vi "Standalone DAQ IO Config UI.vi"() -> ()   [LabVIEW 2022 SP3, in "DAQ.lvclass"]
doc: "Developed by Kevin Thompson\nkevin@thompsonengineering.net\n\nCopyright 2018-2020\nThompson Engineering, LLC"
uses:
  DAQ.lvclass
  DataTypes/TD DI Config--cluster.ctl
  DataTypes/TD DI Task--cluster.ctl
  DataTypes/TD DI Channel--cluster.ctl
  DataTypes/TD DO Config--cluster.ctl
  DataTypes/TD DO Channel--cluster.ctl
  DataTypes/TD AI Config--cluster.ctl
  DataTypes/TD AI Task--cluster.ctl
  DataTypes/TD AI Channel--cluster.ctl
  DataTypes/TD DataValueConversion--cluster.ctl
  DataTypes/TD AI DAQ Type--enum.ctl
  DataTypes/TD AI Force Bridge--cluster.ctl
  DataTypes/TD AO Config--cluster.ctl
  DataTypes/TD AO Channel--cluster.ctl
  DataTypes/TD IO Node Definition--cluster.ctl
panel:
  in  "IO Nodes":T1 {"AO Config"."AO Channels"."Conversion"."ScaleOffset" format="%.3f"; "AO Config"."AO Channels"."Conversion"."MinEngUnit" format="%.3f"; "AO Config"."AO Channels"."Conversion"."MaxEngUnit" format="%.3f"; "AO Config"."AO Channels"."Conversion"."MinSignal" format="%.3f"; "AO Config"."AO Channels"."Conversion"."MaxSignal" format="%.3f"; "AI Config"."AI Tasks"."AI Channels"."Conversion"."ScaleOffset" format="%.3f"; "AI Config"."AI Tasks"."AI Channels"."Conversion"."MinEngUnit" format="%.3f"; "AI Config"."AI Tasks"."AI Channels"."Conversion"."MaxEngUnit" format="%.3f"; "AI Config"."AI Tasks"."AI Channels"."Conversion"."MinSignal" format="%.3f"; "AI Config"."AI Tasks"."AI Channels"."Conversion"."MaxSignal" format="%.3f"; "AI Config"."AI Tasks"."AI Channels"."Terminal Configuration" items=["default"=-1, "RSE"=10083, "NRSE"=10078, "Differential"=10106, "Pseudodifferential"=12529]}
  in  "LoadFile":bool
  in  "Config File":path
  in  "ApplyAll":bool
  out "Error":bool
  in  "Exit":bool
  in  "SaveAll":bool
  out "Tab Control":T15(tab)
  in  "DI Config":T2
  in  "DO Config":T5
  in  "AI Config":T7 {"AI Tasks"."AI Channels"."Force Bridge"."scaling information"."physical units" items=["Newtons"=15875, "Pounds"=15876, "kgf"=15877]; "AI Tasks"."AI Channels"."Force Bridge"."scaling information"."electrical units" items=["Volts/Volt"=15896, "mVolts/Volt"=15897]; "AI Tasks"."AI Channels"."Force Bridge"."bridge information"."voltage excitation source" items=["Internal"=10200, "External"=10167]; "AI Tasks"."AI Channels"."Force Bridge"."bridge information"."bridge configuration" items=["Full Bridge"=10182, "Half Bridge"=10187, "Quarter Bridge"=10270]; "AI Tasks"."AI Channels"."Conversion"."ScaleOffset" format="%.3f"; "AI Tasks"."AI Channels"."Conversion"."MinEngUnit" format="%.3f"; "AI Tasks"."AI Channels"."Conversion"."MaxEngUnit" format="%.3f"; "AI Tasks"."AI Channels"."Conversion"."MinSignal" format="%.3f"; "AI Tasks"."AI Channels"."Conversion"."MaxSignal" format="%.3f"; "AI Tasks"."AI Channels"."Terminal Configuration" items=["default"=-1, "RSE"=10083, "NRSE"=10078, "Differential"=10106, "Pseudodifferential"=12529]}
  in  "AO Config":T13 {"AO Channels"."Conversion"."ScaleOffset" format="%.3f"; "AO Channels"."Conversion"."MinEngUnit" format="%.3f"; "AO Channels"."Conversion"."MaxEngUnit" format="%.3f"; "AO Channels"."Conversion"."MinSignal" format="%.3f"; "AO Channels"."Conversion"."MaxSignal" format="%.3f"}
  in  "ConfigSections":i32(listbox)
  # "D A Q   I O   C O N F I G   U T I L I T Y"
  # "* Application Restart Required"
  # "DI Config"
  # "DO Config"
  # "AI Config"
  # "AO Config"
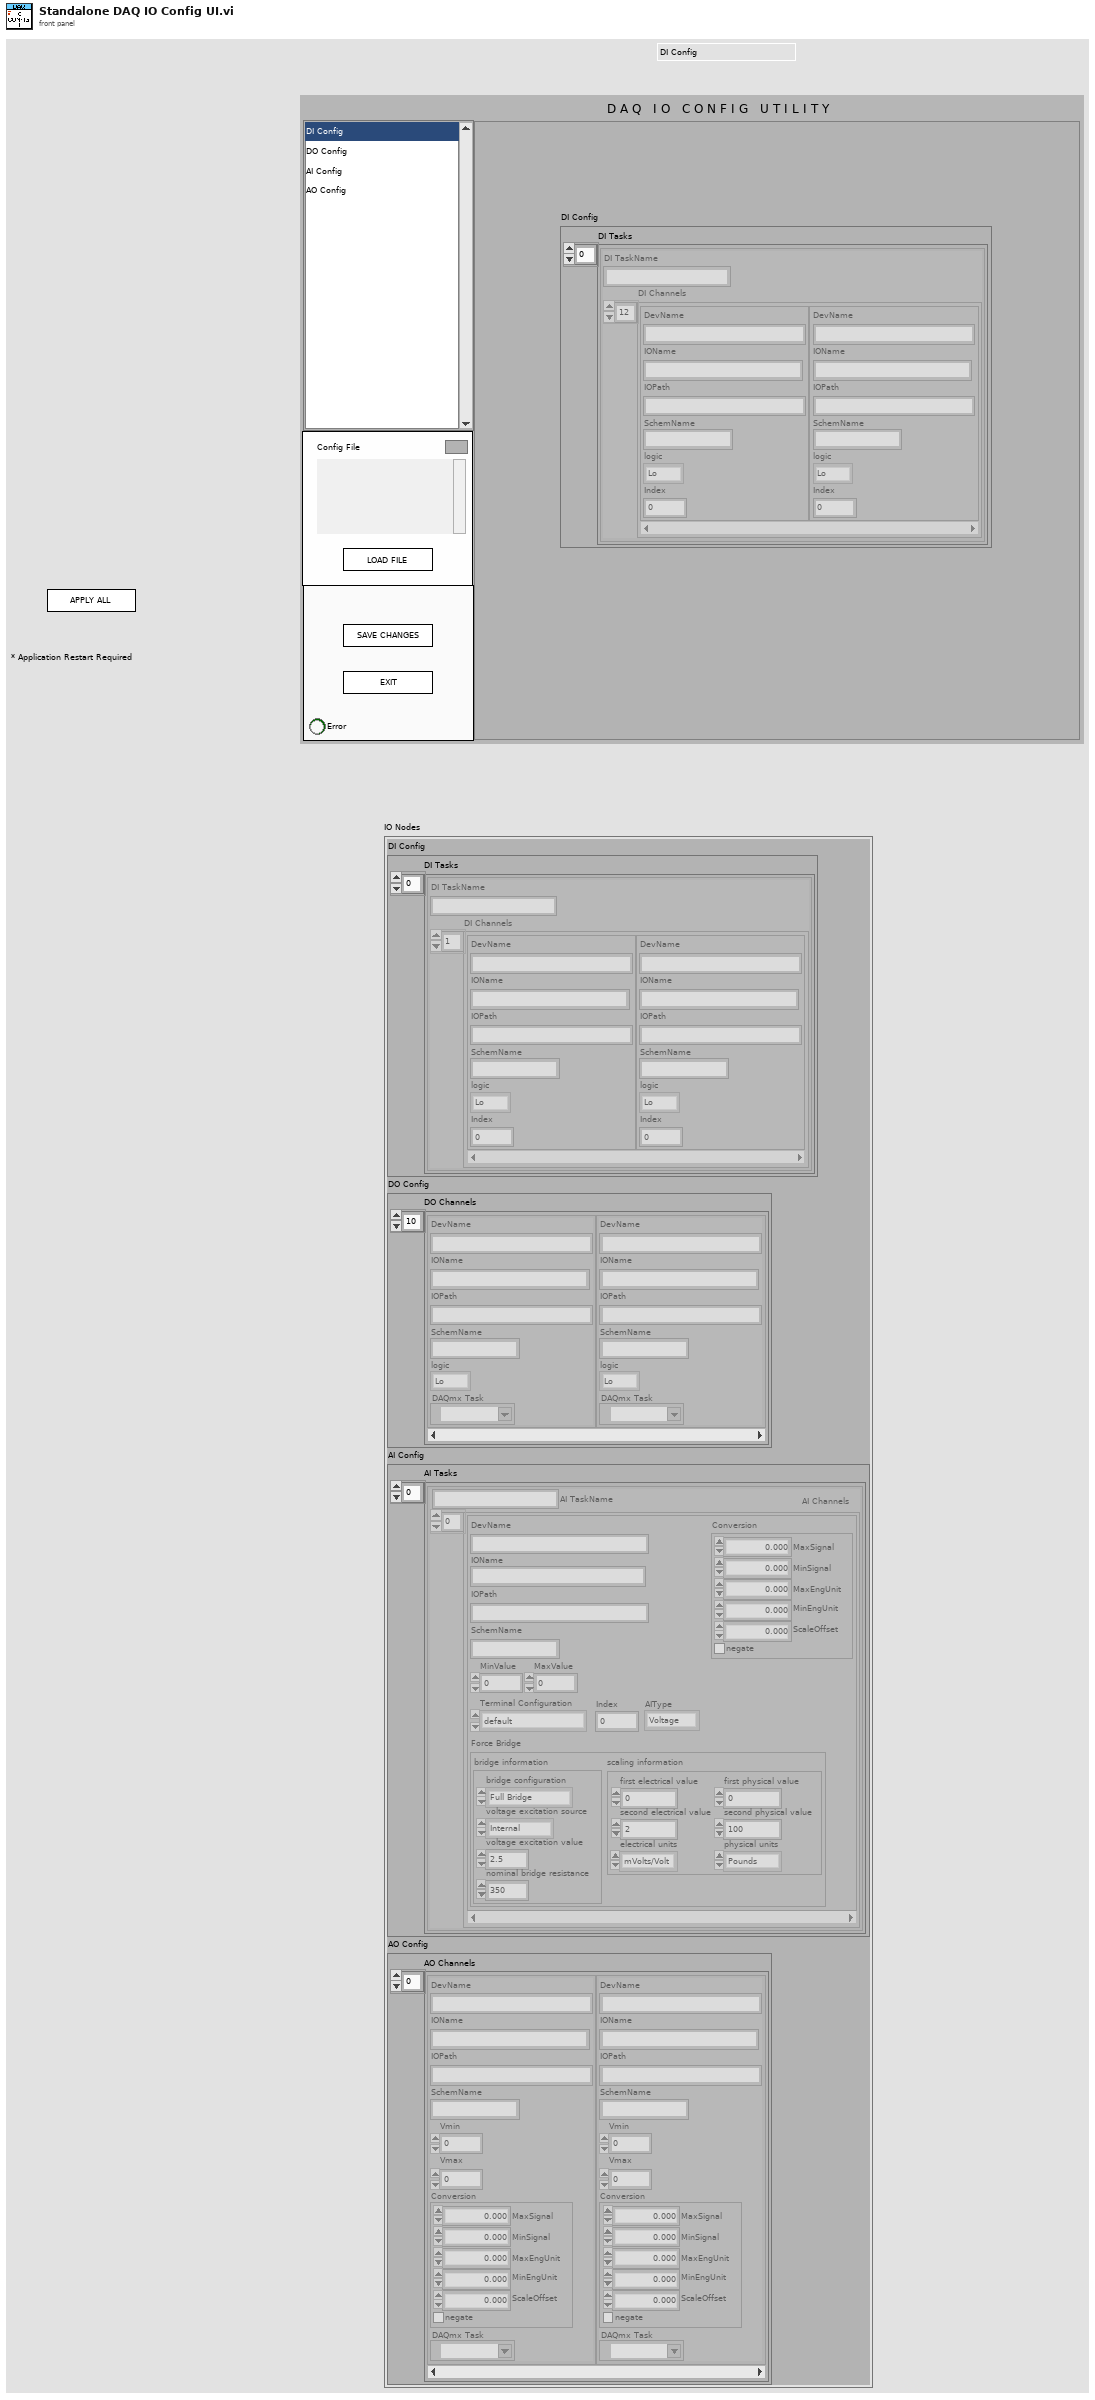
[diagram p1: front panel]
types:
  T1 = typedef "DAQ.lvclass/TD IO Node Definition--cluster.ctl" = cluster{"DI Config":T2, "DO Config":T5, "AI Config":T7, "AO Config":T13}
  T2 = typedef "DAQ.lvclass/TD DI Config--cluster.ctl" = cluster{"DI Tasks":T3[]}
  T3 = typedef "DAQ.lvclass/TD DI Task--cluster.ctl" = cluster{"DI TaskName":string, "DI Channels":T4[]}
  T4 = typedef "DAQ.lvclass/TD DI Channel--cluster.ctl" = cluster{"DevName":string, "IOName":string, "IOPath":string, "SchemName":string, "logic":enum16{"Lo", "Hi"}, "Index":i32}
  T5 = typedef "DAQ.lvclass/TD DO Config--cluster.ctl" = cluster{"DO Channels":T6[]}
  T6 = typedef "DAQ.lvclass/TD DO Channel--cluster.ctl" = cluster{"DevName":string, "IOName":string, "IOPath":string, "SchemName":string, "logic":enum16{"Lo", "Hi"}, "DAQmx Task":refnum<k21>}
  T7 = typedef "DAQ.lvclass/TD AI Config--cluster.ctl" = cluster{"AI Tasks":T8[]}
  T8 = typedef "DAQ.lvclass/TD AI Task--cluster.ctl" = cluster{"AI TaskName":string, "AI Channels":T9[]}
  T9 = typedef "DAQ.lvclass/TD AI Channel--cluster.ctl" = cluster{"DevName":string, "IOName":string, "IOPath":string, "SchemName":string, "MinValue":dbl, "MaxValue":dbl, "Terminal Configuration":i32, "Index":i32, "Conversion":T10, "AIType":T11, "Force Bridge":T12}
  T10 = typedef "DAQ.lvclass/TD DataValueConversion--cluster.ctl" = cluster{"MaxSignal":dbl, "MinSignal":dbl, "MaxEngUnit":dbl, "MinEngUnit":dbl, "ScaleOffset":dbl, "negate":bool}
  T11 = typedef "DAQ.lvclass/TD AI DAQ Type--enum.ctl" = enum16{"Voltage", "Current", "Strain Gage", "Force Bridge"}
  T12 = typedef "DAQ.lvclass/TD AI Force Bridge--cluster.ctl" = cluster{"bridge information":cluster{"bridge configuration":i32, "voltage excitation source":i32, "voltage excitation value":dbl, "nominal bridge resistance":dbl}, "scaling information":cluster{"first electrical value":dbl, "second electrical value":dbl, "electrical units":i32, "first physical value":dbl, "second physical value":dbl, "physical units":i32}}
  T13 = typedef "DAQ.lvclass/TD AO Config--cluster.ctl" = cluster{"AO Channels":T14[]}
  T14 = typedef "DAQ.lvclass/TD AO Channel--cluster.ctl" = cluster{"DevName":string, "IOName":string, "IOPath":string, "SchemName":string, "Vmin":dbl, "Vmax":dbl, "Conversion":T10, "DAQmx Task":refnum<k21>}
  T15 = enum32{"DI Config", "DO Config", "AI Config", "AO Config"}
  T16 = enum32{"Invalid", "Default", "Floating", "Floating/Auto-Hide", "Modal"}
  T17 = enum32{"Invalid", "Standard", "Closed", "Hidden", "Minimized", "Maximized"}
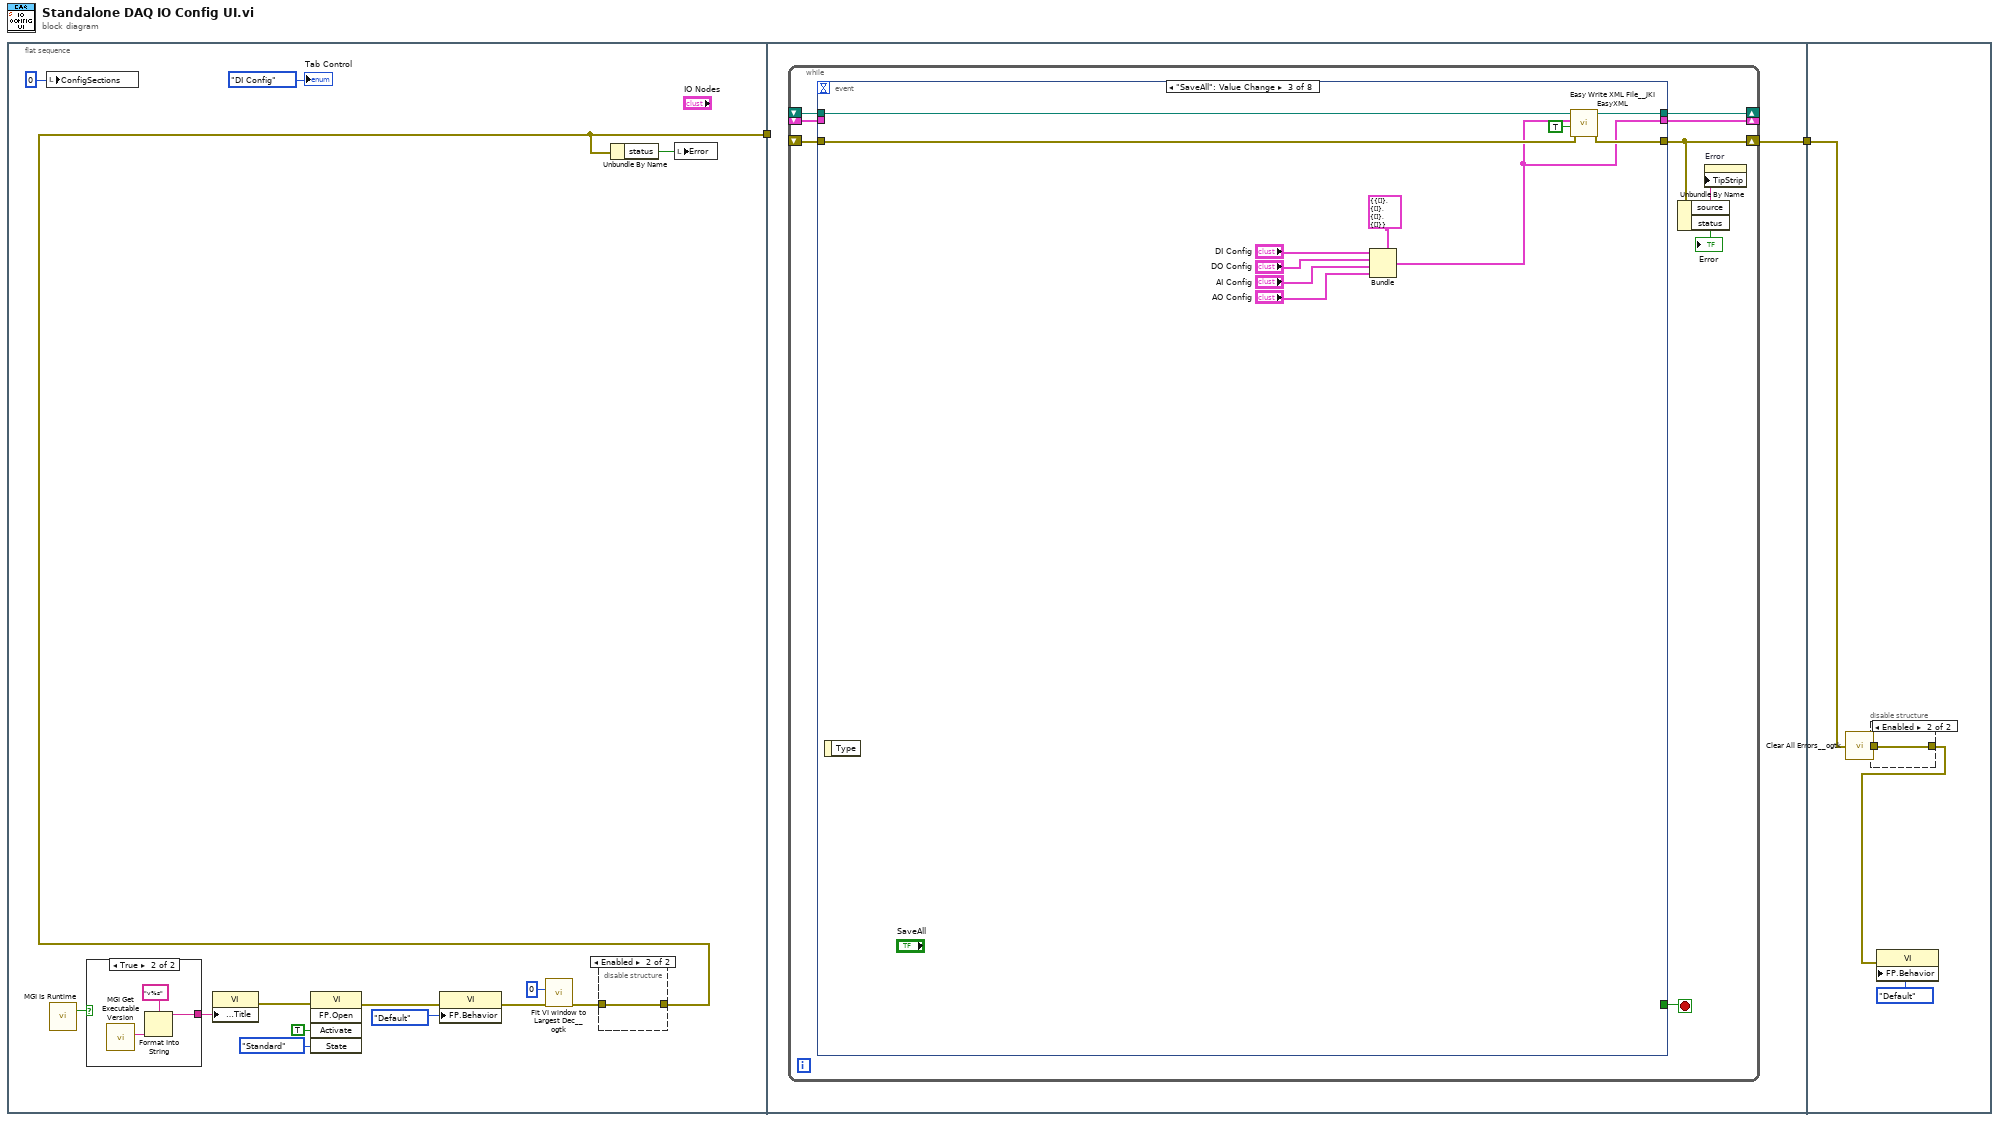
[diagram p0: block diagram]
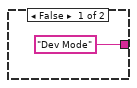
[diagram p2: hidden frame]
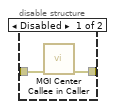
[diagram p3: hidden frame]
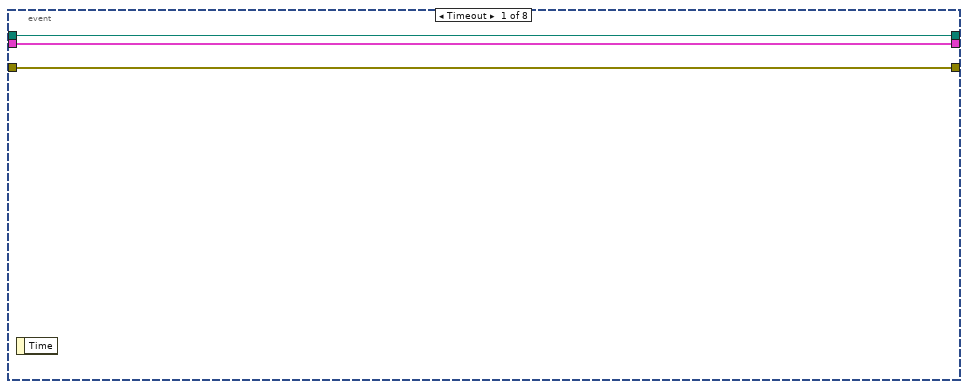
[diagram p4: hidden frame]
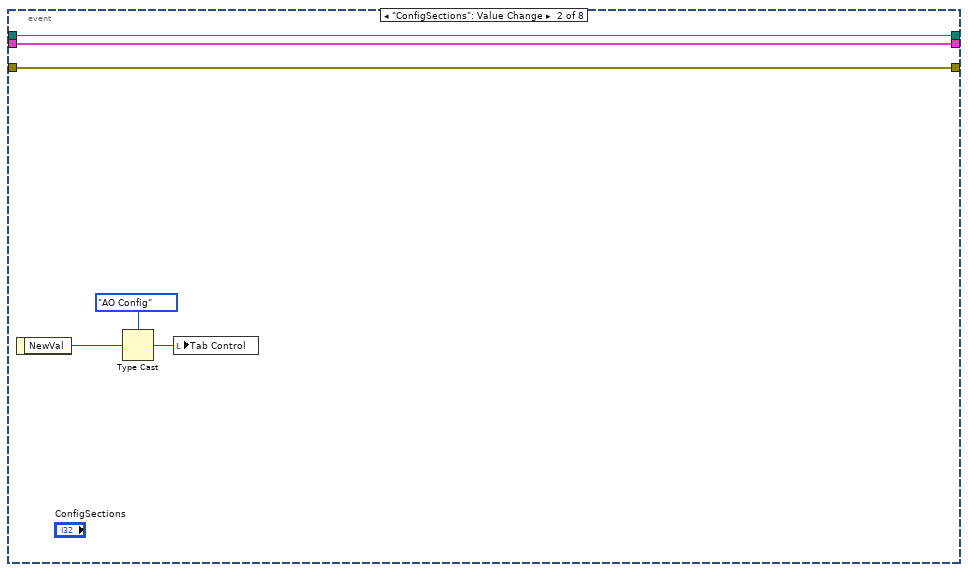
[diagram p5: hidden frame]
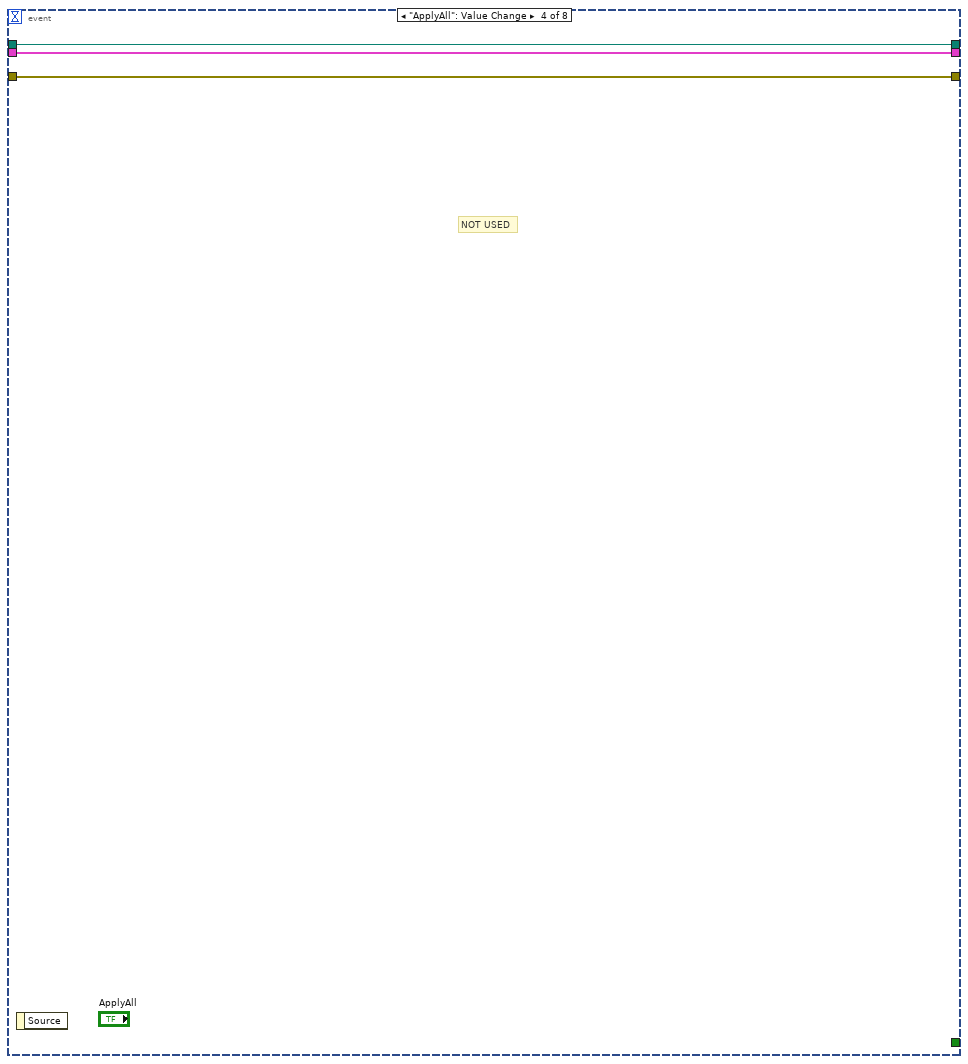
[diagram p6: hidden frame]
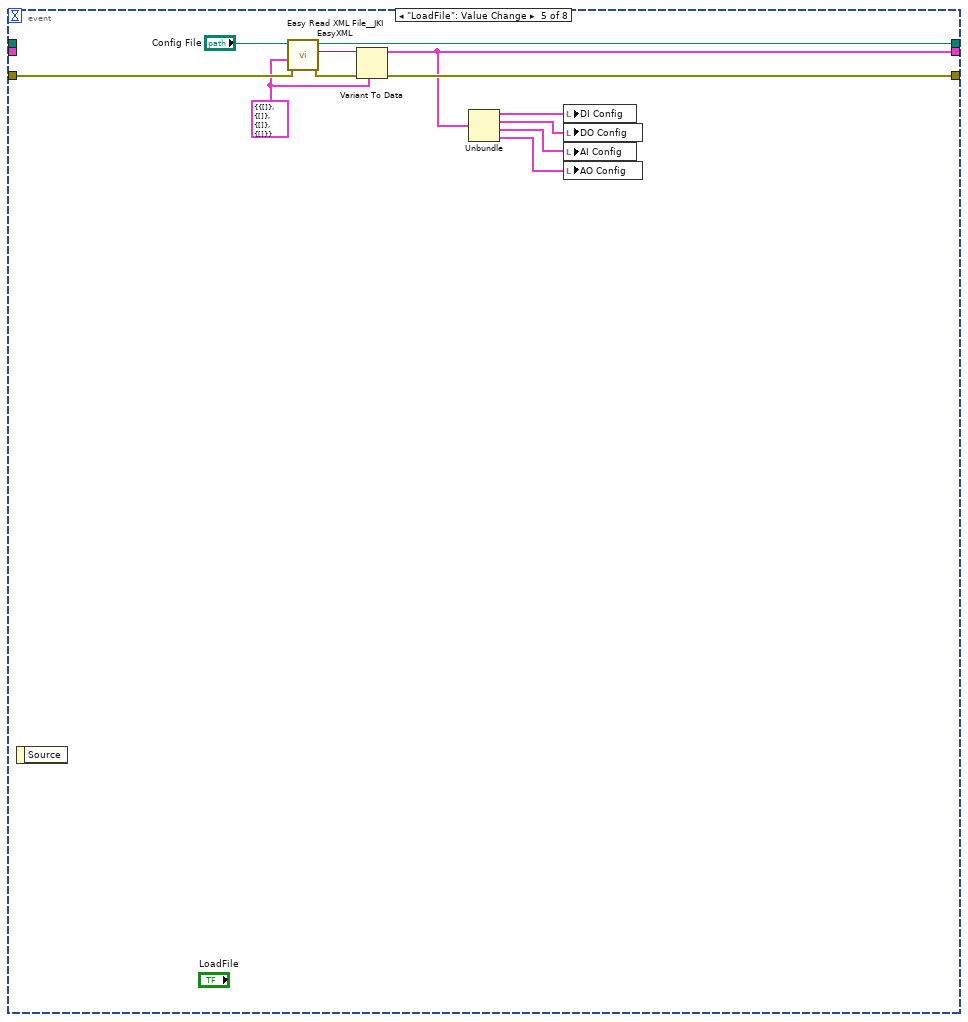
[diagram p7: hidden frame]
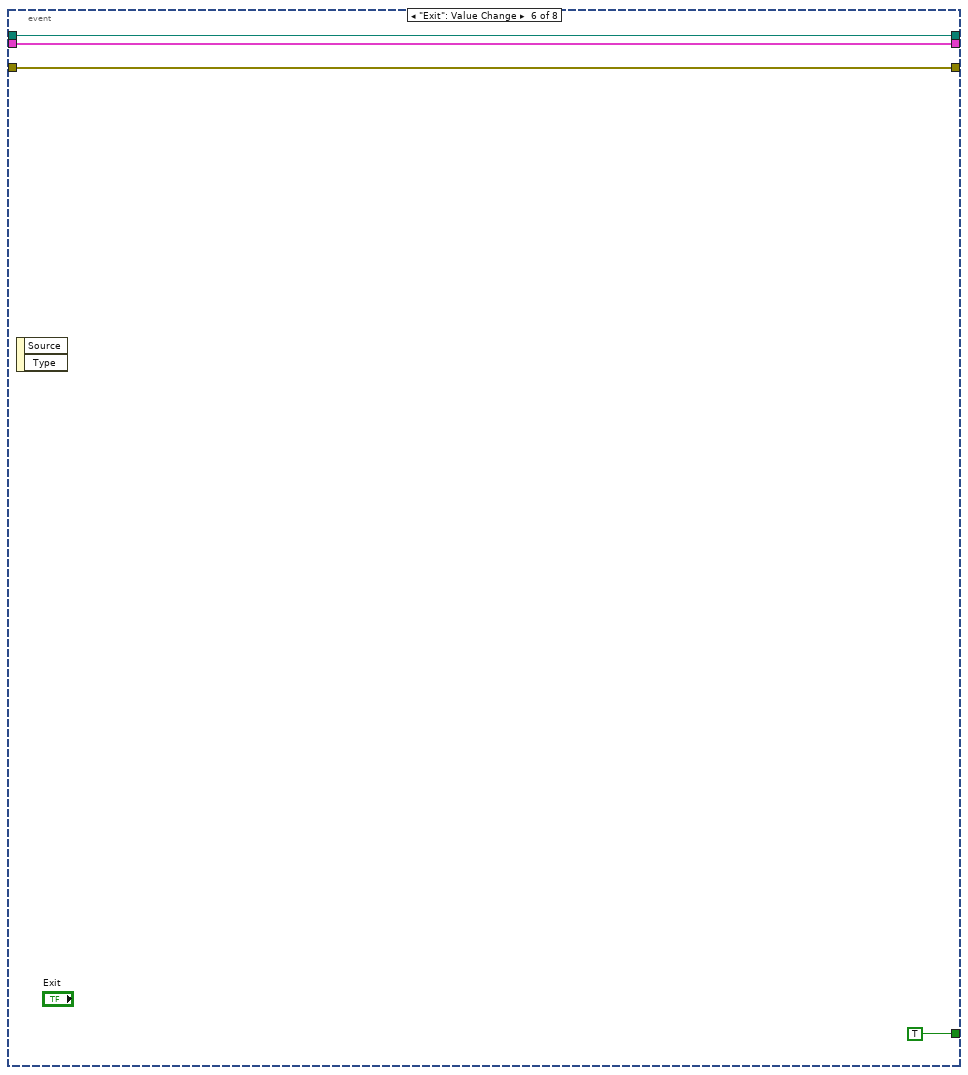
[diagram p8: hidden frame]
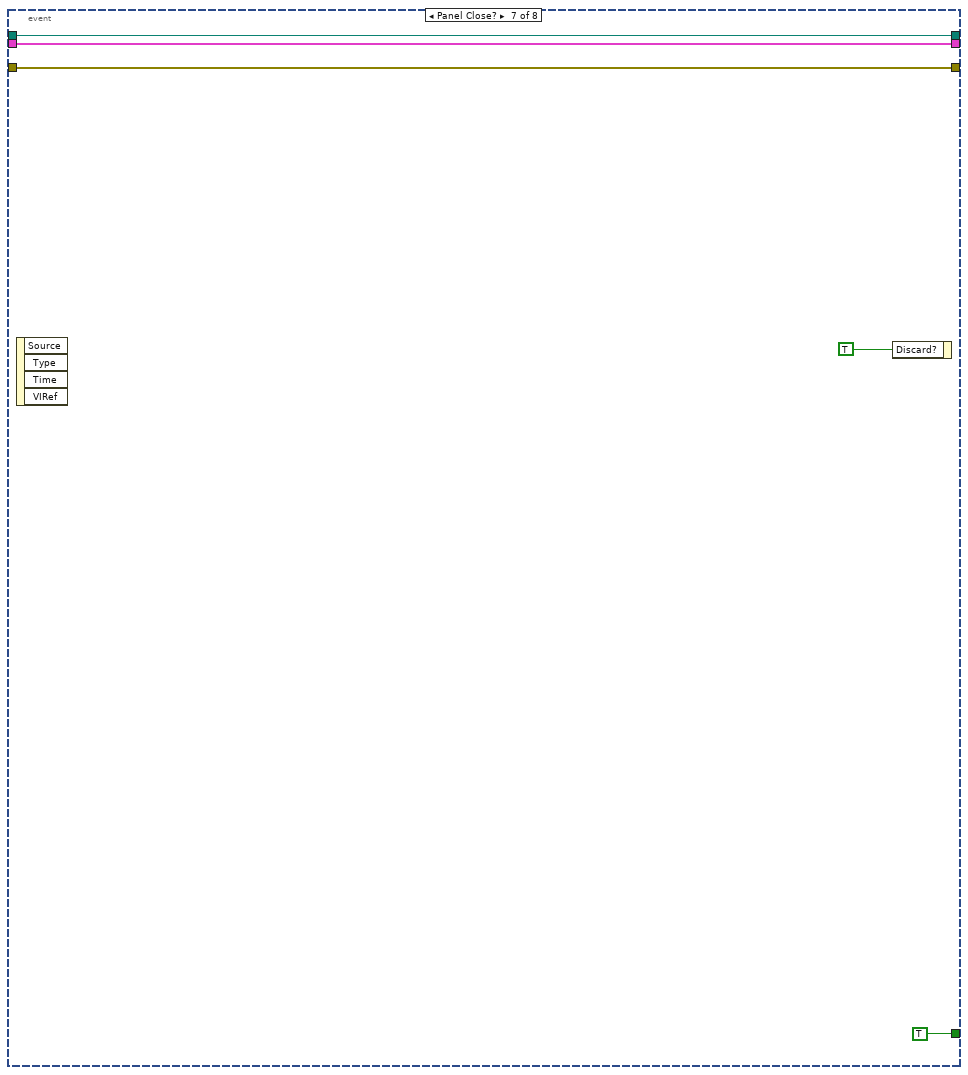
[diagram p9: hidden frame]
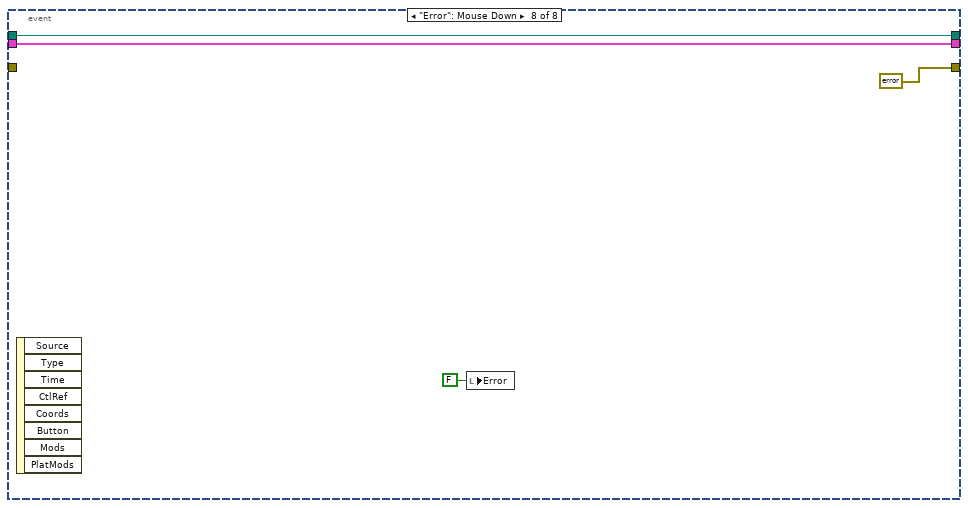
[diagram p10: hidden frame]
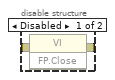
[diagram p11: hidden frame]
diagram:
  n1 = flat-sequence {
    tunnel: [w7] -> w2
    tunnel: w2 -> [_]
    tunnel: [w24] -> w1
    tunnel: w1 -> [w83]
    frame #0 {
      n2 = local write "ConfigSections"(0 ("ConfigSections")) -> ()
      n3 = call <userlib>:"MGI Is Runtime.vi"() -> ("Run Time System?"=w4:bool)  [unwired: 7 in]
      n4 = case shown="True" w4 {
        tunnel: ["Dev Mode" w20] -> w6
        frame False {
        }
        frame True {
          n5 = call <userlib>:"MGI Get Executable Version.vi"() -> ("Version"=w18:string)  [unwired: 7 in]
          n6 = Format Into String(format string="v%s", w18) -> (resulting string=w20:string)  [unwired: 2 in, 1 out]
        }
      }
      n7 = property class="VI"("Front Panel.Title"=w6) -> (error out=w5:errorcluster)  [unwired: 2 in, 1 out]
      n8 = invoke class="VI" method="FP.Open"(error in=w5, "Activate"=TRUE ("Activate?"), "State"=T17."Standard") -> (error out=w11:errorcluster)  [unwired: 2 in, 4 out]
      n9 = property class="VI"(error in=w11, "FP.Behavior"=T16."Default" ("Front Panel Window:Behavior")) -> (error out=w12:errorcluster)  [unwired: 1 in, 1 out]
      n10 = call <userlib>:"Fit VI window to Largest Dec__ogtk.vi"("error in (no error)"=w12, "border spacing (2 px)"=0) -> ("error out"=w9:errorcluster)  [unwired: 4 in, 1 out]
      n11 = disable-structure shown="Enabled" {
        disable-tunnel: w9 -> [w22 w23]
        disable-tunnel: [w21 w23] -> w7
        frame Disabled {
          n12 = call <userlib>:"MGI Center Callee in Caller.vi"("Error In"=w22) -> ("Error Out"=w21:errorcluster)  [unwired: 10 in]
        }
        frame Enabled {
        }
      }
      n13 = Unbundle By Name(w7) -> ("status"=w8:bool)
      n14 = local write "Error"(w8) -> ()
      "Tab Control" <- T15."DI Config" ("Tab Control")
    }
    frame #1 {
      n15 = while {
        shift-right: [w30] -> w24
        shift-left: _ -> [w32]
        shift-right: [w31] -> _
        shift-left: _ -> [w26]
        shift-right: [w28] -> _
        shift-left: _ -> [w27]
        stop <- w33 stop-if-true
        n16 = event shown="[2] \"SaveAll\": Value Change" {
          selector: _ -> [_ _ _ _ _ _ _ _]
          dyn-events: _ -> [_ _ _ _ _ _ _ _]
          timeout: _ -> [_ _ _ _ _ _ _ _]
          tunnel: [_ _ _ _ _ TRUE TRUE _] -> w33
          tunnel: w26 -> [w35 w40 _ w54 _ w70 w74 w81]
          tunnel: w32 -> [w36 w41 w47 w56 w58 w71 w75 _]
          tunnel: [w36 w41 w46 w56 w66 w71 w75 errorcluster {"status"=FALSE, "code"=0, "source"=""} ("input cluster")] -> w30
          tunnel: [w35 w40 w45 w54 w60 w70 w74 w81] -> w31
          tunnel: [w34 w39 w44 w55 w61 w69 w73 w78] -> w28
          tunnel: w27 -> [w34 w39 w48 w55 _ w69 w73 w78]
          event Timeout {
            n17 = event-data() -> ()  [unwired: 1 in, 1 out]
          }
          event "ConfigSections": Value Change {
            n18 = event-data() -> ("NewVal"=w42:i32)  [unwired: 1 in]
            n19 = Type Cast(type=T15."AO Config" ("Tab Control"), x=w42) -> (*(type *) &x=w38:T15)
            n20 = local write "Tab Control"(w38) -> ()
          }
          event "SaveAll": Value Change {
            n21 = event-data() -> ()  [unwired: 1 in, 1 out]
            n22 = Bundle(cluster=T1 {"DI Config"={"DI Tasks"=[]}, "DO Config"={"DO Channels"=[]}, "AI Config"={"AI Tasks"=[]}, "AO Config"={"AO Channels"=[]}} ("IO Nodes"), "DI Config"="DI Config", "DO Config"="DO Config", "AI Config"="AI Config", "AO Config"="AO Config") -> (w45:T1)
            n23 = call <vilib>:"Easy Write XML File__JKI EasyXML.vi"("error in (no error)"=w47, "Overwrite File? (false)"=TRUE, "LabVIEW Data"=w45, "XML File Path"=w48) -> ("error out"=w46:errorcluster, "XML File Path (duplicate)"=w44:path)  [unwired: 6 in]
          }
          event "ApplyAll": Value Change {
            # "NOT USED"
            n24 = event-data() -> ()  [unwired: 1 in, 1 out]
          }
          event "LoadFile": Value Change {
            w57 = T1 {"DI Config"={"DI Tasks"=[]}, "DO Config"={"DO Channels"=[]}, "AI Config"={"AI Tasks"=[]}, "AO Config"={"AO Channels"=[]}} ("IO Nodes")
            n25 = event-data() -> ()  [unwired: 1 in, 1 out]
            n26 = call <vilib>:"Easy Read XML File__JKI EasyXML.vi"("error in (no error)"=w58, "LabVIEW Data (Type)"=w57, "XML File Path"="Config File") -> ("error out"=w59:errorcluster, "LabVIEW Data"=w68:variant, "XML File Path (duplicate)"=w61:path)  [unwired: 6 in]
            n27 = Variant To Data(error in=w59, type=w57, Variant=w68) -> (data=w60:T1, error out=w66:errorcluster)
            n28 = Unbundle(w60) -> ("DI Config"=w65:T2, "DO Config"=w64:T5, "AI Config"=w63:T7, "AO Config"=w62:T13)
            n29 = local write "DI Config"(w65) -> ()
            n30 = local write "DO Config"(w64) -> ()
            n31 = local write "AI Config"(w63) -> ()
            n32 = local write "AO Config"(w62) -> ()
          }
          event "Exit": Value Change {
            n33 = event-data() -> ()  [unwired: 1 in, 2 out]
          }
          event Panel Close? {
            n34 = event-data() -> ()  [unwired: 1 in, 4 out]
            n35 = event-data("Discard?"=TRUE) -> ()  [unwired: 1 in, 1 out]
          }
          event "Error": Mouse Down {
            n36 = event-data() -> ()  [unwired: 1 in, 8 out]
            n37 = local write "Error"(FALSE ("Error")) -> ()
          }
        }
        n38 = Unbundle By Name(w30) -> ("source"=w25:string, "status"=→"Error":bool)
        n39 = property on="Error" class="Bool (strict)"("TipStrip"=w25) -> ()  [unwired: 2 in, 2 out]
      }
    }
    frame #2 {
      n40 = call <userlib>:"Clear All Errors__ogtk.vi"("Error In"=w83) -> ("Error Out"=w82:errorcluster)  [unwired: 3 in]
      n41 = disable-structure shown="Enabled" {
        disable-tunnel: [w87 w88] -> w84
        disable-tunnel: w82 -> [w86 w88]
        frame Disabled {
          n42 = invoke class="VI" method="FP.Close"(error in=w86) -> (error out=w87:errorcluster)  [unwired: 2 in, 2 out]
        }
        frame Enabled {
        }
      }
      n43 = property class="VI"(error in=w84, "FP.Behavior"=T16."Default" ("Front Panel Window:Behavior")) -> ()  [unwired: 1 in, 2 out]
    }
  }
